vi "StopOrError.vi"(8 "error in":errorcluster, 9 "StoppedIn":bool) -> (0 "error_out":errorcluster, 1 "!Error":bool, 4 "StoppedOut":bool)   [LabVIEW 2013]
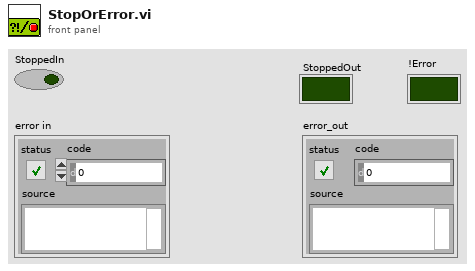
[diagram p1: front panel]
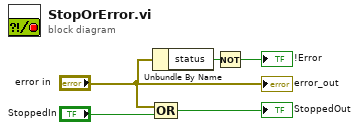
[diagram p0: block diagram]
diagram:
  n1 = Unbundle By Name("error in") -> ("status"=w2:bool)
  n2 = Compound Arithmetic op=OR("error in", "StoppedIn") -> (→"StoppedOut":bool)
  n3 = Not(x=w2) -> (.not. x?=→"!Error":bool)
  "error_out" <- "error in"
